vi "registrarOffset.vi"(8 "error in (no error)":errorcluster, 10 "Offsets":i64[](array[numeric]), 11 "semaphore":T1) -> (0 "error out":errorcluster, 3 "semaphore out":T1)   [LabVIEW 2015]
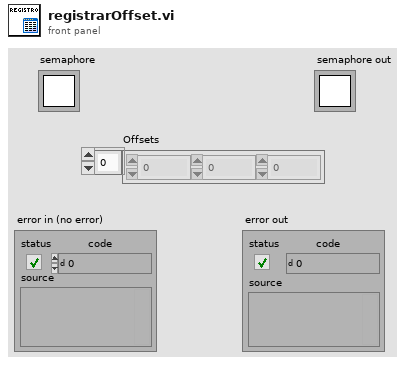
[diagram p1: front panel]
types:
  T1 = typedef "Semaphore RefNum" = refnum<k1>
  T2 = enum16{"open", "open or create", "create or replace", "create", "open (read-only)"}
  T3 = cluster{"tdms control out":refnum<k34>, "tdms historial out":refnum<k34>, "tdms sinc out":refnum<k34>}
  T4 = cluster{"tdms file out":refnum<k34>, "tdms file out":refnum<k34>, "tdms file out":refnum<k34>}
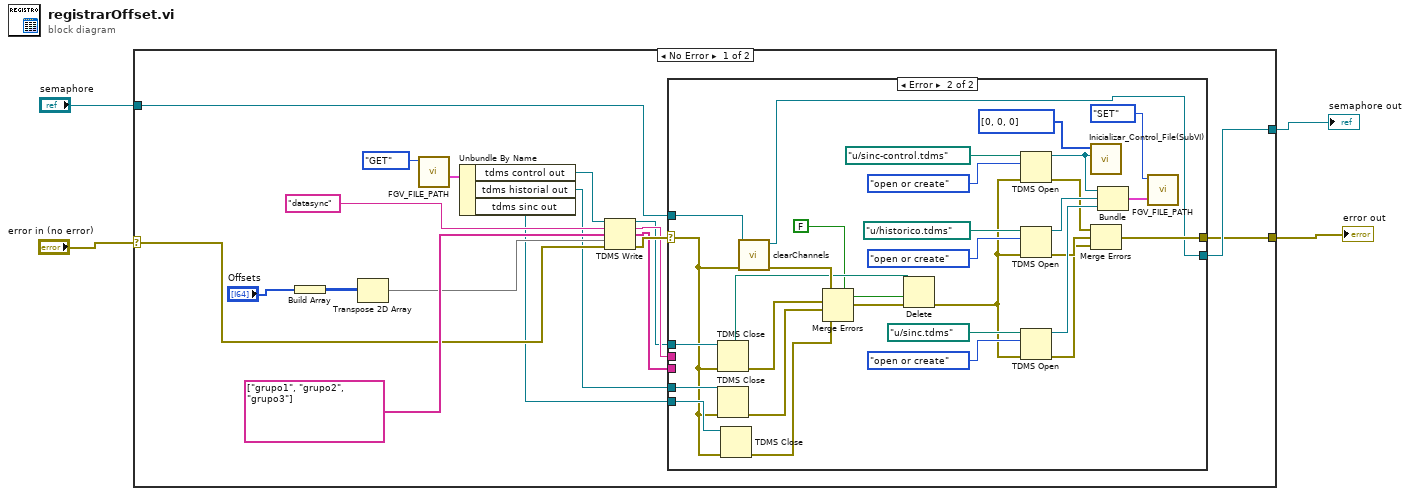
[diagram p0: block diagram]
diagram:
  n1 = case shown="No Error" "error in (no error)" {
    selector: "error in (no error)" -> [w17 w56]
    tunnel: [w10 w56] -> w3
    tunnel: [w11 w55] -> w2
    tunnel: "semaphore" -> [w12 w55]
    frame No Error {
      n2 = Build Array("Offsets") -> (w19:i64[][])
      n3 = Transpose 2D Array(2D array=w19) -> (transposed array=w18:i64[][])
      n4 = call "FGV_FILE_PATH.vi"("Function"=enum16{"GET", "SET"}."GET") -> ("Data Out"=w15:T3)  [unwired: 10 in]
      n5 = Unbundle By Name(w15) -> ("tdms control out"=w14:refnum<k34>, "tdms historial out"=w6:refnum<k34>, "tdms sinc out"=w5:refnum<k34>)
      n6 = TDMS Write(0:w14, 5:"datasync" ("group name in"), 7:string[] ["grupo1", "grupo2", "grupo3"], 9:w18, 11:w17) -> (4:w7:refnum<k34>, 6:w8:string, 8:w9:string[], 15:w13:errorcluster)  [unwired: 1 in]
      n7 = case shown="Error" w13 {
        selector: w13 -> [w23 w34]
        tunnel: w12 -> [w24 w54]
        tunnel: [w24 w32] -> w11
        tunnel: [w23 w37] -> w10
        tunnel: w9 -> [_ _]
        tunnel: w8 -> [_ _]
        tunnel: w7 -> [_ w53]
        tunnel: w6 -> [_ w36]
        tunnel: w5 -> [_ w35]
        frame No Error {
        }
        frame Error {
          n8 = TDMS Close(8:w34, 11:w53) -> (0:w31:errorcluster, 3:w28:path)
          n9 = TDMS Close(8:w34, 11:w36) -> (0:w30:errorcluster)  [unwired: 1 out]
          n10 = TDMS Close(8:w34, 11:w35) -> (0:w29:errorcluster)  [unwired: 1 out]
          n11 = call "clearChannels.vi"("error in"=w34, "semaphore"=w54) -> ("error out"=w33:errorcluster, "semaphore out"=w32:T1)  [unwired: 8 in]
          n12 = Merge Errors(w33, w31, w30, w29) -> (w26:errorcluster)
          n13 = Delete(path (use dialog)=w28, confirm (F)=FALSE, error in=w26) -> (error out=w25:errorcluster)  [unwired: 2 in, 2 out]
          n14 = TDMS Open(8:w25, 10:T2."open or create" ("operation (0:open)"), 11:path "u:/sinc-control.tdms" ("file path")) -> (0:w40:errorcluster, 3:w49:refnum<k34>)  [unwired: 4 in]
          n15 = TDMS Open(8:w25, 10:T2."open or create" ("operation (0:open)"), 11:path "u:/historico.tdms" ("file path")) -> (0:w39:errorcluster, 3:w47:refnum<k34>)  [unwired: 4 in]
          n16 = TDMS Open(8:w25, 10:T2."open or create" ("operation (0:open)"), 11:path "u:/sinc.tdms" ("file path")) -> (0:w38:errorcluster, 3:w43:refnum<k34>)  [unwired: 4 in]
          n17 = call "Inicializar_Control_File(SubVI).vi"("tdms file"=w49, "Offsets"=i64[] [0, 0, 0]) -> ()  [unwired: 9 in, 1 out]
          n18 = Merge Errors(w40, w39, w38) -> (w37:errorcluster)
          n19 = Bundle("tdms file out"=w49, "tdms file out"=w47, "tdms file out"=w43) -> (w42:T4)  [unwired: 1 in]
          n20 = call "FGV_FILE_PATH.vi"("Data In"=w42, "Function"=enum16{"GET", "SET"}."SET") -> ()  [unwired: 9 in, 1 out]
        }
      }
    }
    frame Error {
    }
  }
  "error out" <- w3
  "semaphore out" <- w2
